vi "Color Sensor(SubVI).vi"() -> ()   [LabVIEW 2017]
uses:
  <vilib>/functionblocks/Edge Detection/Edge Detect/Edge Detect.vi
  <vilib>/functionblocks/FB Core/FB Core.xnode
  <vilib>/functionblocks/NI_FunctionBlock Libraries.lvlib
panel:
  out "Waveform Chart":dbl(graph)
  out "Numeric":dbl
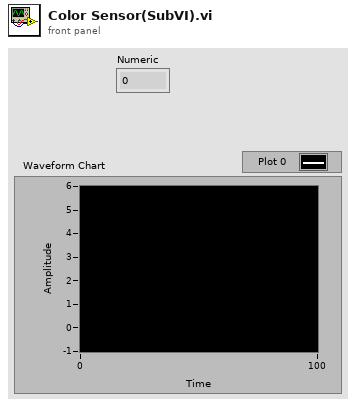
[diagram p1: front panel]
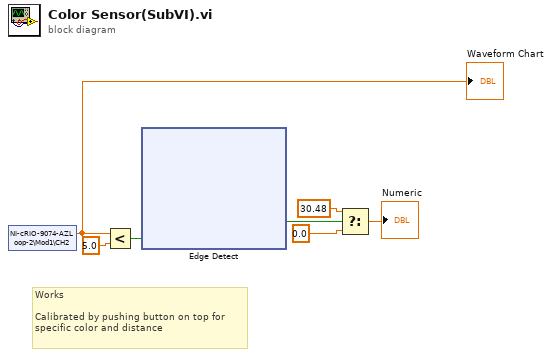
[diagram p0: block diagram]
diagram:
  # "Works\n\nCalibrated by pushing button on top for\nspecific color and distance"
  n1 = shared-variable "NI-cRIO-9074-AZLoop-2\\Mod1\\CH2"() -> (w1:dbl)  [unwired: 1 in, 1 out]
  "Waveform Chart" <- w1
  n2 = Less?(x=w1, y=5.0) -> (x < y?=w6:bool)
  n3 = xnode "Edge Detect"("input 1"=w6) -> ("output"=w5:bool)  [unwired: 2 in, 1 out]
  n4 = Select(t=30.48, s=w5, f=0.0) -> (s? t:f=→"Numeric":dbl)
